vi "Snake Case to Standard.vi"(8 "error in (no error)":errorcluster, 11 "Input String":string) -> (0 "error out":errorcluster, 3 "Output String":string)   [LabVIEW 2015, in "Case Manipulation.lvlib"]
doc: "Introduction:\nWe often remove the spaces between words because programs of different sorts reserve the space (‘ ’) character for special purposes. Because the space character is reserved, we cannot use it to represent a concept that we express in our human language with multiple words.\nSnake Case:\nThis style, when capitalized, is often used as a convention in declaring constants in many languages. When lower cased, it is used conventionally in declaring database field names."
uses:
  Case Manipulation.lvlib
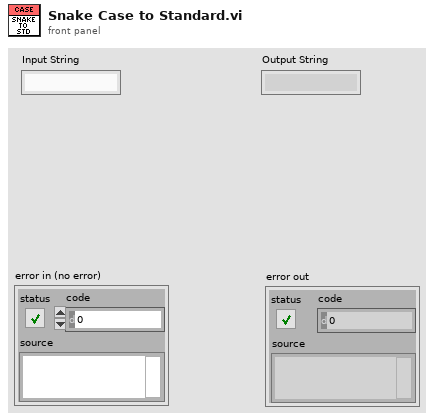
[diagram p1: front panel]
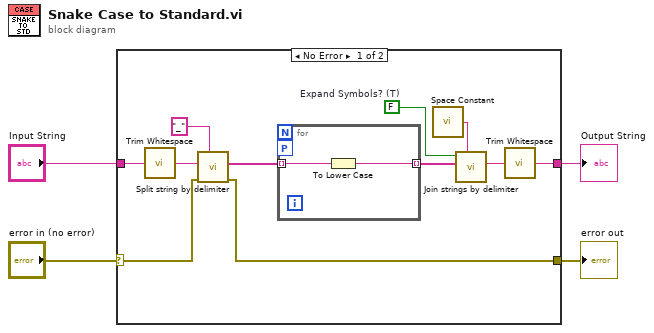
[diagram p0: block diagram]
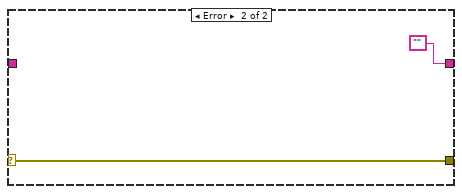
[diagram p2: hidden frame]
diagram:
  n1 = case shown="No Error" "error in (no error)" {
    selector: "error in (no error)" -> [w9 w18]
    tunnel: [w8 w18] -> w2
    tunnel: [w11 ""] -> w1
    tunnel: "Input String" -> [w15 _]
    frame No Error {
      w5 = FALSE  # Expand Symbols? (T)
      n2 = call <vilib>:"Trim Whitespace.vi"("string"=w15) -> ("trimmed string"=w10:string)  [unwired: 1 in]
      n3 = call "Split string by delimiter.vi"("Delimiter"="_", "error in (no error)"=w9, "String In"=w10) -> ("error out"=w8:errorcluster, "String Array Out"=w7:string[])  [unwired: 7 in]
      n4 = for {
        tunnel: w7 -> [w17] mode=indexing
        tunnel: [w16] -> w14 mode=indexing
        workers-P: _ -> [_]
        n5 = To Lower Case(string=w17) -> (all lower case string=w16:string)
      }
      n6 = call <vilib>:"Space Constant.vi"() -> ("String"=w13:string)
      n7 = call "Join strings by delimiter.vi"("Delimiter"=w13, "Strings []"=w14, "Expand Symbols? (T)"=w5) -> ("String Out"=w12:string)  [unwired: 8 in]
      n8 = call <vilib>:"Trim Whitespace.vi"("string"=w12) -> ("trimmed string"=w11:string)  [unwired: 1 in]
    }
    frame Error {
    }
  }
  "error out" <- w2
  "Output String" <- w1
